vi "Lex Set Delimiter Example.vi"(8 "Error In":errorcluster) -> (0 "Error Out":errorcluster)   [LabVIEW 2018, in "Tests.lvlib" / "Lexer.lvlib"]
uses:
  Lexer.lvlib
  src/Toolkit/Low-Level/Tokens/Text/Text.lvclass
  src/Toolkit/Low-Level/Tokens/EscapedVariable/EscapedVariable.lvclass
  src/Toolkit/Low-Level/Tokens/SetDelimiter/SetDelimiter.lvclass
  src/Toolkit/Low-Level/Support/Lex String.vi
  <vilib>/Utility/LVClass/Get LV Class Name.vi
  src/Toolkit/Low-Level/Tokens/Contentable/Contentable.lvclass
  src/Toolkit/Low-Level/Tokens/Keyable/Keyable.lvclass
  <vilib>/addons/_JKI Toolkits/Caraya/classes/Test/Test.lvclass
  <vilib>/addons/_JKI Toolkits/Caraya/classes/Assert/Assert.lvclass
  Tests.lvlib
  src/Toolkit/Toolkit.lvlib
  src/Toolkit/Low-Level/Tokens/Token/Token.lvclass
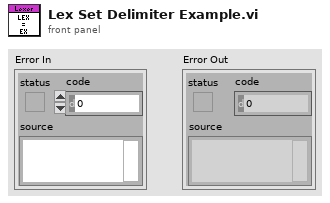
[diagram p1: front panel]
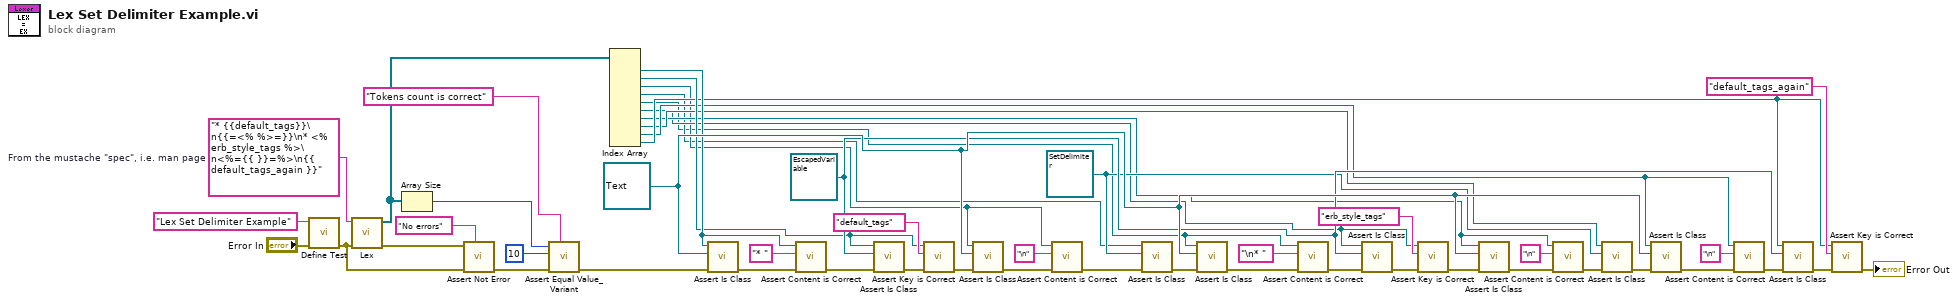
[diagram p0: block diagram]
diagram:
  w11 = refnum<class "SetDelimiter.lvclass"> refnum ("Toolkit.lvlib:Tokens.lvlib:SetDelimiter.lvclass")
  w21 = refnum<class "EscapedVariable.lvclass"> refnum ("Mustache.lvlib:Tokens.lvlib:EscapedVariable.lvclass")
  w26 = refnum<class "Text.lvclass"> refnum ("Mustache.lvlib:Tokens.lvlib:Text.lvclass")
  w18 = "* {{default_tags}}\n{{=<% %>=}}\n* <% erb_style_tags %>\n<%={{ }}=%>\n{{ default_tags_again }}"  # From the mustache "spec", i.e. man page
  n1 = call <vilib>:"Define Test.vi"("error in (no error)"="Error In", "Label (VI Title)"="Lex Set Delimiter Example") -> ("error out"=w19:errorcluster)  [unwired: 9 in]
  n2 = call-poly "Lex.vi"("Error In"=w19, "Input"=w18) -> ("Error Out"=w49:errorcluster, "Tokens"=w43:refnum<class "Token.lvclass">[])  [unwired: 8 in]
  n3 = Array Size(array=w43) -> (size(s)=w45:i32)
  n4 = call <vilib>:"Assert Not Error.vi"("Label"="No errors", "error in (no error)"=w19, "Not Error?"=w49) -> ("error out"=w47:errorcluster)  [unwired: 8 in]
  n5 = call <vilib>:"Assert Equal Value_Variant.vi"("Label"="Tokens count is correct", "error in (no error)"=w47, "Y"=10 ("size(s)"), "X"=w45) -> ("error out"=w42:errorcluster)  [unwired: 7 in]
  n6 = Index Array(array=w43) -> (element #1=w17:refnum<class "Token.lvclass">, element #2=w16:refnum<class "Token.lvclass">, element #3=w3:refnum<class "Token.lvclass">, element #4=w2:refnum<class "Token.lvclass">, element #5=w1:refnum<class "Token.lvclass">, element #6=w8:refnum<class "Token.lvclass">, element #7=w9:refnum<class "Token.lvclass">, element #8=w10:refnum<class "Token.lvclass">, element #9=w14:refnum<class "Token.lvclass">, element #10=w15:refnum<class "Token.lvclass">)  [unwired: 10 in]
  n7 = call "Assert Is Class.vi"("Error In"=w42, "Expected"=w26, "Actual"=w17) -> ("Error Out"=w41:errorcluster)  [unwired: 8 in]
  n8 = call "Assert Content is Correct.vi"("Error In"=w41, "Expected"="* ", "Token"=w17) -> ("Error Out"=w39:errorcluster)  [unwired: 8 in]
  n9 = call "Assert Is Class.vi"("Error In"=w39, "Expected"=w21, "Actual"=w16) -> ("Error Out"=w38:errorcluster)  [unwired: 8 in]
  n10 = call "Assert Key is Correct.vi"("Error In"=w38, "Expected"="default_tags", "Token"=w16) -> ("Error Out"=w4:errorcluster)  [unwired: 8 in]
  n11 = call "Assert Is Class.vi"("Error In"=w4, "Expected"=w26, "Actual"=w3) -> ("Error Out"=w36:errorcluster)  [unwired: 8 in]
  n12 = call "Assert Content is Correct.vi"("Error In"=w36, "Expected"="\n", "Token"=w3) -> ("Error Out"=w6:errorcluster)  [unwired: 8 in]
  n13 = call "Assert Is Class.vi"("Error In"=w6, "Expected"=w11, "Actual"=w2) -> ("Error Out"=w5:errorcluster)  [unwired: 8 in]
  n14 = call "Assert Is Class.vi"("Error In"=w5, "Expected"=w26, "Actual"=w1) -> ("Error Out"=w7:errorcluster)  [unwired: 8 in]
  n15 = call "Assert Content is Correct.vi"("Error In"=w7, "Expected"="\n* ", "Token"=w1) -> ("Error Out"=w33:errorcluster)  [unwired: 8 in]
  n16 = call "Assert Is Class.vi"("Error In"=w33, "Expected"=w21, "Actual"=w8) -> ("Error Out"=w32:errorcluster)  [unwired: 8 in]
  n17 = call "Assert Key is Correct.vi"("Error In"=w32, "Expected"="erb_style_tags", "Token"=w8) -> ("Error Out"=w30:errorcluster)  [unwired: 8 in]
  n18 = call "Assert Is Class.vi"("Error In"=w30, "Expected"=w26, "Actual"=w9) -> ("Error Out"=w29:errorcluster)  [unwired: 8 in]
  n19 = call "Assert Content is Correct.vi"("Error In"=w29, "Expected"="\n", "Token"=w9) -> ("Error Out"=w13:errorcluster)  [unwired: 8 in]
  n20 = call "Assert Is Class.vi"("Error In"=w13, "Expected"=w11, "Actual"=w10) -> ("Error Out"=w12:errorcluster)  [unwired: 8 in]
  n21 = call "Assert Is Class.vi"("Error In"=w12, "Expected"=w26, "Actual"=w14) -> ("Error Out"=w27:errorcluster)  [unwired: 8 in]
  n22 = call "Assert Content is Correct.vi"("Error In"=w27, "Expected"="\n", "Token"=w14) -> ("Error Out"=w24:errorcluster)  [unwired: 8 in]
  n23 = call "Assert Is Class.vi"("Error In"=w24, "Expected"=w21, "Actual"=w15) -> ("Error Out"=w23:errorcluster)  [unwired: 8 in]
  n24 = call "Assert Key is Correct.vi"("Error In"=w23, "Expected"="default_tags_again", "Token"=w15) -> ("Error Out"=→"Error Out":errorcluster)  [unwired: 8 in]
